vi "DisplayJson.vi"(11 "JSON String In":string="[{\"version\":\"1.0.0\",\"header\":{\"creationDate\":\"2022-06-03T00:00:00\",\"remarks\":\"\",\"serialNumber\":\"98172\",\"productNumber\":\"123021.1804\",\"productType\":\"PAA-9L\",\"pressureType\":2,\"productSeries\":\"9L\",\"compensatedTemperatureRange\":{\"min\":-10.0,\"max\":80.0,\"unit\":4},\"compensatedPressureRange\":{\"min\":0.0,\"max\":0.35,\"unit\":3},\"electricSupply\":{\"magnitude\":1.0,\"unit\":18},\"orderNumber\":9990266,\"orderPosition\":3,\"orderTargetDispatchDate\":\"2022-06-02T00:00:00+00:00\",\"customerName\":\"DemoData Inc.\",\"customerNumber\":12345678,\"customerOrderNumber\":\"Cust-9990266-123\",\"customerReferenceNumber\":\"\",\"customerProductT...") -> ()   [LabVIEW 2017] (continued)
arget\":{\"pressure\":{\"magnitude\":0.03,\"unit\":3},\"temperature\":{\"magnitude\":80.0,\"unit\":4}},\"environment\":{\"pressure\":{\"magnitude\":0.0300006,\"unit\":3},\"temperature\":{\"magnitude\":79.9513,\"unit\":4},\"supply\":{\"magnitude\":1.0,\"unit\":18}},\"raw\":{\"signal\":{\"magnitude\":18.112910598,\"unit\":22},\"bridgeResistance\":{\"magnitude\":4053.922893,\"unit\":28}},\"compensated\":{\"mathematicalModels\":{\"MM0123\":{\"pressure\":{\"output\":{\"magnitude\":0.0300226,\"unit\":3},\"error\":{\"magnitude\":0.0062805229,\"unit\":7}},\"temperature\":{\"output\":{\"magnitude\":80.0426,\"unit\":4},\"error\":{\"magnitude\":0.091262449,\"unit\":4}}}}}},{\"reference\":\"F_12300_XX_0000098765\",\"environmentTarget\":{\"pressure\":{\"magnitude\":0.11,\"unit\":3},\"temperature\":{\"magnitude\":80.0,\"unit\":4}},\"environment\":{\"pressure\":{\"magnitude\":0.110004,\"unit\":3},\"temperature\":{\"magnitude\":79.9513,\"unit\":4},\"supply\":{\"magnitude\":1.0,\"unit\":18}},\"raw\":{\"signal\":{\"magnitude\":30.219828489,\"unit\":22},\"bridgeResistance\":{\"magnitude\":4049.2092548,\"unit\":28}},\"compensated\":{\"mathematicalModels\":{\"MM0123\":{\"pressure\":{\"output\":{\"magnitude\":0.109956,\"unit\":3},\"error\":{\"magnitude\":-0.013573045,\"unit\":7}},\"temperature\":{\"output\":{\"magnitude\":80.0465,\"unit\":4},\"error\":{\"magnitude\":0.095120343,\"unit\":4}}}}}},{\"reference\":\"F_12300_XX_0000098765\",\"environmentTarget\":{\"pressure\":{\"magnitude\":0.19,\"unit\":3},\"temperature\":{\"magnitude\":80.0,\"unit\":4}},\"environment\":{\"pressure\":{\"magnitude\":0.189994,\"unit\":3},\"temperature\":{\"magnitude\":79.9513,\"unit\":4},\"supply\":{\"magnitude\":1.0,\"unit\":18}},\"raw\":{\"signal\":{\"magnitude\":42.312978657,\"unit\":22},\"bridgeResistance\":{\"magnitude\":4044.5861667,\"unit\":28}},\"compensated\":{\"mathematicalModels\":{\"MM0123\":{\"pressure\":{\"output\":{\"magnitude\":0.189999,\"unit\":3},\"error\":{\"magnitude\":0.0015625619,\"unit\":7}},\"temperature\":{\"output\":{\"magnitude\":80.0544,\"unit\":4},\"error\":{\"magnitude\":0.10309475,\"unit\":4}}}}}},{\"reference\":\"F_12300_XX_0000098765\",\"environmentTarget\":{\"pressure\":{\"magnitude\":0.27,\"unit\":3},\"temperature\":{\"magnitude\":80.0,\"unit\":4}},\"environment\":{\"pressure\":{\"magnitude\":0.270001,\"unit\":3},\"temperature\":{\"magnitude\":79.9513,\"unit\":4},\"supply\":{\"magnitude\":1.0,\"unit\":18}},\"raw\":{\"signal\":{\"magnitude\":54.374135615,\"unit\":22},\"bridgeResistance\":{\"magnitude\":4040.0065092,\"unit\":28}},\"compensated\":{\"mathematicalModels\":{\"MM0123\":{\"pressure\":{\"output\":{\"magnitude\":0.270039,\"unit\":3},\"error\":{\"magnitude\":0.01094065,\"unit\":7}},\"temperature\":{\"output\":{\"magnitude\":80.0614,\"unit\":4},\"error\":{\"magnitude\":0.11007026,\"unit\":4}}}}}},{\"reference\":\"F_12300_XX_0000098765\",\"environmentTarget\":{\"pressure\":{\"magnitude\":0.35,\"unit\":3},\"temperature\":{\"magnitude\":80.0,\"unit\":4}},\"environment\":{\"pressure\":{\"magnitude\":0.349998,\"unit\":3},\"temperature\":{\"magnitude\":79.9513,\"unit\":4},\"supply\":{\"magnitude\":1.0,\"unit\":18}},\"raw\":{\"signal\":{\"magnitude\":66.389691162,\"unit\":22},\"bridgeResistance\":{\"magnitude\":4035.4744179,\"unit\":28}},\"compensated\":{\"mathematicalModels\":{\"MM0123\":{\"pressure\":{\"output\":{\"magnitude\":0.349978,\"unit\":3},\"error\":{\"magnitude\":-0.0056827473,\"unit\":7}},\"temperature\":{\"output\":{\"magnitude\":80.0671,\"unit\":4},\"error\":{\"magnitude\":0.11580255,\"unit\":4}}}}}}]},{\"version\":\"1.0.0\",\"header\":{\"creationDate\":\"2022-06-03T00:00:00\",\"remarks\":\"\",\"serialNumber\":\"98062\",\"productNumber\":\"123021.1804\",\"productType\":\"PAA-9L\",\"pressureType\":2,\"productSeries\":\"9L\",\"compensatedTemperatureRange\":{\"min\":-10.0,\"max\":80.0,\"unit\":4},\"compensatedPressureRange\":{\"min\":0.0,\"max\":0.35,\"unit\":3},\"electricSupply\":{\"magnitude\":1.0,\"unit\":18},\"orderNumber\":9990266,\"orderPosition\":3,\"orderTargetDispatchDate\":\"2022-06-02T00:00:00+00:00\",\"customerName\":\"DemoData Inc.\",\"customerNumber\":12345678,\"customerOrderNumber\":\"Cust-9990266-123\",\"customerReferenceNumber\":\"\",\"customerProductType\":\"123021-1804 Rev.AA\"},\"compensationMethods\":{\"mathematicalModels\":{\"MM0123\":{\"modelType\":\"MM0123\",\"productNumber\":\"000000.0000\",\"compensatedTemperatureRange\":{\"min\":-10.0,\"max\":80.0,\"unit\":4},\"compensatedPressureRange\":{\"min\":0.0,\"max\":0.35,\"unit\":3},\"electricSupply\":{\"magnitude\":1.0,\"unit\":18},\"parts\":{\"pressure\":{\"inputs\":[\"Sig\",\"R\"],\"output\":\"P\",\"description\":\"P = f(Sig,R)\",\"coefficients\":[[4.24498616654,-0.00434870646169,1.65645526915E-06,-2.82503980815E-10,1.80574905609E-14],[-0.136709021669,0.000147073956199,-5.65029989332E-08,9.64480704004E-12,-6.18362859613E-16],[4.40289191256E-05,-2.40851139109E-08,1.82732990774E-12,9.42409772251E-16,-1.43118016035E-19]]},\"temperature\":{\"inputs\":[\"R\",\"Sig\"],\"output\":\"T\",\"description\":\"T = f(R,Sig)\",\"coefficients\":[[-8429.66589229,19.4262004834,-0.189958165455],[8.28473398531,-0.0200345175176,0.000205816813801],[-0.00311774743246,7.78515900293E-06,-8.35927190864E-08],[5.30811398776E-07,-1.34715910968E-09,1.50785989149E-11],[-3.40839033724E-11,8.75216679413E-14,-1.01901855741E-15]]}}}}},\"measurements\":[{\"reference\":\"F_12300_XX_0000098765\",\"environmentTarget\":{\"pressure\":{\"magnitude\":0.03,\"unit\":3},\"temperature\":{\"magnitude\":-10.0,\"unit\":4}},\"environment\":{\"pressure\":{\"magnitude\":0.030006,\"unit\":3},\"temperature\":{\"magnitude\":-10.7286,\"unit\":4},\"supply\":{\"magnitude\":1.0,\"unit\":18}},\"raw\":{\"signal\":{\"magnitude\":16.167899598,\"unit\":22},\"bridgeResistance\":{\"magnitude\":3278.97235,\"unit\":28}},\"compensated\":{\"mathematicalModels\":{\"MM0123\":{\"pressure\":{\"output\":{\"magnitude\":0.0300194,\"unit\":3},\"error\":{\"magnitude\":0.003820477,\"unit\":7}},\"temperature\":{\"output\":{\"magnitude\":-10.8437,\"unit\":4},\"error\":{\"magnitude\":-0.11506924,\"unit\":4}}}}}},{\"reference\":\"F_12300_XX_0000098765\",\"environmentTarget\":{\"pressure\":{\"magnitude\":0.11,\"unit\":3},\"temperature\":{\"magnitude\":-10.0,\"unit\":4}},\"environment\":{\"pressure\":{\"magnitude\":0.110008,\"unit\":3},\"temperature\":{\"magnitude\":-10.7286,\"unit\":4},\"supply\":{\"magnitude\":1.0,\"unit\":18}},\"raw\":{\"signal\":{\"magnitude\":28.175220871,\"unit\":22},\"bridgeResistance\":{\"magnitude\":3274.3397417,\"unit\":28}},\"compensated\":{\"mathematicalModels\":{\"MM0123\":{\"pressure\":{\"output\":{\"magnitude\":0.109973,\"unit\":3},\"error\":{\"magnitude\":-0.010122702,\"unit\":7}},\"temperature\":{\"output\":{\"magnitude\":-10.8462,\"unit\":4},\"error\":{\"magnitude\":-0.11753739,\"unit\":4}}}}}},{\"reference\":\"F_12300_XX_0000098765\",\"environmentTarget\":{\"pressure\":{\"magnitude\":0.19,\"unit\":3},\"temperature\":{\"magnitude\":-10.0,\"unit\":4}},\"environment\":{\"pressure\":{\"magnitude\":0.190005,\"unit\":3},\"temperature\":{\"magnitude\":-10.7286,\"unit\":4},\"supply\":{\"magnitude\":1.0,\"unit\":18}},\"raw\":{\"signal\":{\"magnitude\":40.141769614,\"unit\":22},\"bridgeResistance\":{\"magnitude\":3269.8255782,\"unit\":28}},\"compensated\":{\"mathematicalModels\":{\"MM0123\":{\"pressure\":{\"output\":{\"magnitude\":0.190013,\"unit\":3},\"error\":{\"magnitude\":0.0022029902,\"unit\":7}},\"temperature\":{\"output\":{\"magnitude\":-10.8464,\"unit\":4},\"error\":{\"magnitude\":-0.11774787,\"unit\":4}}}}}},{\"reference\":\"F_12300_XX_0000098765\",\"environmentTarget\":{\"pressure\":{\"magnitude\":0.27,\"unit\":3},\"temperature\":{\"magnitude\":-10.0,\"unit\":4}},\"environment\":{\"pressure\":{\"magnitude\":0.270008,\"unit\":3},\"temperature\":{\"magnitude\":-10.7286,\"unit\":4},\"supply\":{\"magnitude\":1.0,\"unit\":18}},\"raw\":{\"signal\":{\"magnitude\":52.052658113,\"unit\":22},\"bridgeResistance\":{\"magnitude\":3265.4291158,\"unit\":28}},\"compensated\":{\"mathematicalModels\":{\"MM0123\":{\"pressure\":{\"output\":{\"magnitude\":0.270043,\"unit\":3},\"error\":{\"magnitude\":0.0098634549,\"unit\":7}},\"temperature\":{\"output\":{\"magnitude\":-10.8462,\"unit\":4},\"error\":{\"magnitude\":-0.11753424,\"unit\":4}}}}}},{\"reference\":\"F_12300_XX_0000098765\",\"environmentTarget\":{\"pressure\":{\"magnitude\":0.35,\"unit\":3},\"temperature\":{\"magnitude\":-10.0,\"unit\":4}},\"environment\":{\"pressure\":{\"magnitude\":0.350001,\"unit\":3},\"temperature\":{\"magnitude\":-10.7286,\"unit\":4},\"supply\":{\"magnitude\":1.0,\"unit\":18}},\"raw\":{\"signal\":{\"magnitude\":63.897706655,\"unit\":22},\"bridgeResistance\":{\"magnitude\":3261.1318651,\"unit\":28}},\"compensated\":{\"mathematicalModels\":{\"MM0123\":{\"pressure\":{\"output\":{\"magnitude\":0.349995,\"unit\":3},\"error\":{\"magnitude\":-0.0017233202,\"unit\":7}},\"temperature\":{\"output\":{\"magnitude\":-10.8497,\"unit\":4},\"error\":{\"magnitude\":-0.12110753,\"unit\":4}}}}}},{\"reference\":\"F_12300_XX_0000098765\",\"environmentTarget\":{\"pressure\":{\"magnitude\":0.03,\"unit\":3},\"temperature\":{\"magnitude\":0.0,\"unit\":4}},\"environment\":{\"pressure\":{\"magnitude\":0.0300032,\"unit\":3},\"temperature\":{\"magnitude\":-0.629962,\"unit\":4},\"supply\":{\"magnitude\":1.0,\"unit\":18}},\"raw\":{\"signal\":{\"magnitude\":16.623830617,\"unit\":22},\"bridgeResistance\":{\"magnitude\":3347.8748473,\"unit\":28}},\"compensated\":{\"mathematicalModels\":{\"MM0123\":{\"pressure\":{\"output\":{\"magnitude\":0.0300186,\"unit\":3},\"error\":{\"magnitude\":0.0044065173,\"unit\":7}},\"temperature\":{\"output\":{\"magnitude\":-0.743773,\"unit\":4},\"error\":{\"magnitude\":-0.11381103,\"unit\":4}}}}}},{\"reference\":\"F_12300_XX_0000098765\",\"environmentTarget\":{\"pressure\":{\"magnitude\":0.11,\"unit\":3},\"temperature\":{\"magnitude\":0.0,\"unit\":4}},\"environment\":{\"pressure\":{\"magnitude\":0.110005,\"unit\":3},\"temperature\":{\"magnitude\":-0.629962,\"unit\":4},\"supply\":{\"magnitude\":1.0,\"unit\":18}},\"raw\":{\"signal\":{\"magnitude\":28.598303294,\"unit\":22},\"bridgeResistance\":{\"magnitude\":3343.279329,\"unit\":28}},\"compensated\":{\"mathematicalModels\":{\"MM0123\":{\"pressure\":{\"output\":{\"magnitude\":0.109969,\"unit\":3},\"error\":{\"magnitude\":-0.010291145,\"unit\":7}},\"temperature\":{\"output\":{\"magnitude\":-0.747222,\"unit\":4},\"error\":{\"magnitude\":-0.11726057,\"unit\":4}}}}}},{\"reference\":\"F_12300_XX_0000098765\",\"environmentTarget\":{\"pressure\":{\"magnitude\":0.19,\"unit\":3},\"temperature\":{\"magnitude\":0.0,\"unit\":4}},\"environment\":{\"pressure\":{\"magnitude\":0.190007,\"unit\":3},\"temperature\":{\"magnitude\":-0.629962,\"unit\":4},\"supply\":{\"magnitude\":1.0,\"unit\":18}},\"raw\":{\"signal\":{\"magnitude\":40.534914808,\"unit\":22},\"bridgeResistance\":{\"magnitude\":3338.7917735,\"unit\":28}},\"compensated\":{\"mathematicalModels\":{\"MM0123\":{\"pressure\":{\"output\":{\"magnitude\":0.190008,\"unit\":3},\"error\":{\"magnitude\":0.00028916783,\"unit\":7}},\"temperature\":{\"output\":{\"magnitude\":-0.74744,\"unit\":4},\"error\":{\"magnitude\":-0.11747789,\"unit\":4}}}}}},{\"reference\":\"F_12300_XX_0000098765\",\"environmentTarget\":{\"pressure\":{\"magnitude\":0.27,\"unit\":3},\"temperature\":{\"magnitude\":0.0,\"unit\":4}},\"environment\":{\"pressure\":{\"magnitude\":0.269999,\"unit\":3},\"temperature\":{\"magnitude\":-0.629962,\"unit\":4},\"supply\":{\"magnitude\":1.0,\"unit\":18}},\"raw\":{\"signal\":{\"magnitude\":52.415254612,\"unit\":22},\"bridgeResistance\":{\"magnitude\":3334.362312,\"unit\":28}},\"compensated\":{\"mathematicalModels\":{\"MM0123\":{\"pressure\":{\"output\":{\"magnitude\":0.270016,\"unit\":3},\"error\":{\"magnitude\":0.0047200097,\"unit\":7}},\"temperature\":{\"output\":{\"magnitude\":-0.752861,\"unit\":4},\"error\":{\"magnitude\":-0.12289898,\"unit\":4}}}}}},{\"reference\":\"F_12300_XX_0000098765\",\"environmentTarget\":{\"pressure\":{\"magnitude\":0.35,\"unit\":3},\"temperature\":{\"magnitude\":0.0,\"unit\":4}},\"environment\":{\"pressure\":{\"magnitude\":0.350007,\"unit\":3},\"temperature\":{\"magnitude\":-0.629962,\"unit\":4},\"supply\":{\"magnitude\":1.0,\"unit\":18}},\"raw\":{\"signal\":{\"magnitude\":64.236943105,\"unit\":22},\"bridgeResistance\":{\"magnitude\":3330.0559863,\"unit\":28}},\"compensated\":{\"mathematicalModels\":{\"MM0123\":{\"pressure\":{\"output\":{\"magnitude\":0.349973,\"unit\":3},\"error\":{\"magnitude\":-0.0097175853,\"unit\":7}},\"temperature\":{\"output\":{\"magnitude\":-0.754914,\"unit\":4},\"error\":{\"magnitude\":-0.12495178,\"unit\":4}}}}}},{\"reference\":\"F_12300_XX_0000098765\",\"environmentTarget\":{\"pressure\":{\"magnitude\":0.03,\"unit\":3},\"temperature\":{\"magnitude\":20.0,\"unit\":4}},\"environment\":{\"pressure\":{\"magnitude\":0.0299948,\"unit\":3},\"temperature\":{\"magnitude\":19.5509,\"unit\":4},\"supply\":{\"magnitude\":1.0,\"unit\":18}},\"raw\":{\"signal\":{\"magnitude\":17.582834891,\"unit\":22},\"bridgeResistance\":{\"magnitude\":3503.2026052,\"unit\":28}},\"compensated\":{\"mathematicalModels\":{\"MM0123\":{\"pressure\":{\"output\":{\"magnitude\":0.0300099,\"unit\":3},\"error\":{\"magnitude\":0.004308579,\"unit\":7}},\"temperature\":{\"output\":{\"magnitude\":19.5413,\"unit\":4},\"error\":{\"magnitude\":-0.009571961,\"unit\":4}}}}}},{\"reference\":\"F_12300_XX_0000098765\",\"environmentTarget\":{\"pressure\":{\"magnitude\":0.11,\"unit\":3},\"temperature\":{\"magnitude\":20.0,\"unit\":4}},\"environment\":{\"pressure\":{\"magnitude\":0.109994,\"unit\":3},\"temperature\":{\"magnitude\":19.5509,\"unit\":4},\"supply\":{\"magnitude\":1.0,\"unit\":18}},\"raw\":{\"signal\":{\"magnitude\":29.550682095,\"unit\":22},\"bridgeResistance\":{\"magnitude\":3498.58799,\"unit\":28}},\"compensated\":{\"mathematicalModels\":{\"MM0123\":{\"pressure\":{\"output\":{\"magnitude\":0.109966,\"unit\":3},\"error\":{\"magnitude\":-0.008013191,\"unit\":7}},\"temperature\":{\"output\":{\"magnitude\":19.5351,\"unit\":4},\"error\":{\"magnitude\":-0.015746182,\"unit\":4}}}}}},{\"reference\":\"F_12300_XX_0000098765\",\"environmentTarget\":{\"pressure\":{\"magnitude\":0.19,\"unit\":3},\"temperature\":{\"magnitude\":20.0,\"unit\":4}},\"environment\":{\"pressure\":{\"magnitude\":0.19,\"unit\":3},\"temperature\":{\"magnitude\":19.5509,\"unit\":4},\"supply\":{\"magnitude\":1.0,\"unit\":18}},\"raw\":{\"signal\":{\"magnitude\":41.485081135,\"unit\":22},\"bridgeResistance\":{\"magnitude\":3494.0870258,\"unit\":28}},\"compensated\":{\"mathematicalModels\":{\"MM0123\":{\"pressure\":{\"output\":{\"magnitude\":0.190006,\"unit\":3},\"error\":{\"magnitude\":0.0016759146,\"unit\":7}},\"temperature\":{\"output\":{\"magnitude\":19.5339,\"unit\":4},\"error\":{\"magnitude\":-0.016980767,\"unit\":4}}}}}},{\"reference\":\"F_12300_XX_0000098765\",\"environmentTarget\":{\"pressure\":{\"magnitude\":0.27,\"unit\":3},\"temperature\":{\"magnitude\":20.0,\"unit\":4}},\"environment\":{\"pressure\":{\"magnitude\":0.269991,\"unit\":3},\"temperature\":{\"magnitude\":19.5509,\"unit\":4},\"supply\":{\"magnitude\":1.0,\"unit\":18}},\"raw\":{\"signal\":{\"magnitude\":53.37070629,\"unit\":22},\"bridgeResistance\":{\"magnitude\":3489.6192286,\"unit\":28}},\"compensated\":{\"mathematicalModels\":{\"MM0123\":{\"pressure\":{\"output\":{\"magnitude\":0.270031,\"unit\":3},\"error\":{\"magnitude\":0.011358778,\"unit\":7}},\"temperature\":{\"output\":{\"magnitude\":19.5271,\"unit\":4},\"error\":{\"magnitude\":-0.0237925,\"unit\":4}}}}}},{\"reference\":\"F_12300_XX_0000098765\",\"environmentTarget\":{\"pressure\":{\"magnitude\":0.35,\"unit\":3},\"temperature\":{\"magnitude\":20.0,\"unit\":4}},\"environment\":{\"pressure\":{\"magnitude\":0.350002,\"unit\":3},\"temperature\":{\"magnitude\":19.5509,\"unit\":4},\"supply\":{\"magnitude\":1.0,\"unit\":18}},\"raw\":{\"signal\":{\"magnitude\":65.203270025,\"unit\":22},\"bridgeResistance\":{\"magnitude\":3485.2648231,\"unit\":28}},\"compensated\":{\"mathematicalModels\":{\"MM0123\":{\"pressure\":{\"output\":{\"magnitude\":0.350008,\"unit\":3},\"error\":{\"magnitude\":0.0016539591,\"unit\":7}},\"temperature\":{\"output\":{\"magnitude\":19.5242,\"unit\":4},\"error\":{\"magnitude\":-0.026645966,\"unit\":4}}}}}},{\"reference\":\"F_12300_XX_0000098765\",\"environmentTarget\":{\"pressure\":{\"magnitude\":0.03,\"unit\":3},\"temperature\":{\"magnitude\":40.0,\"unit\":4}},\"environment\":{\"pressure\":{\"magnitude\":0.0300084,\"unit\":3},\"temperature\":{\"magnitude\":39.7284,\"unit\":4},\"supply\":{\"magnitude\":1.0,\"unit\":18}},\"raw\":{\"signal\":{\"magnitude\":18.627411057,\"unit\":22},\"bridgeResistance\":{\"magnitude\":3679.0495206,\"unit\":28}},\"compensated\":{\"mathematicalModels\":{\"MM0123\":{\"pressure\":{\"output\":{\"magnitude\":0.0300252,\"unit\":3},\"error\":{\"magnitude\":0.004810232,\"unit\":7}},\"temperature\":{\"output\":{\"magnitude\":39.7236,\"unit\":4},\"error\":{\"magnitude\":-0.0048319572,\"unit\":4}}}}}},{\"reference\":\"F_12300_XX_0000098765\",\"environmentTarget\":{\"pressure\":{\"magnitude\":0.11,\"unit\":3},\"temperature\":{\"magnitude\":40.0,\"unit\":4}},\"environment\":{\"pressure\":{\"magnitude\":0.110007,\"unit\":3},\"temperature\":{\"magnitude\":39.7284,\"unit\":4},\"supply\":{\"magnitude\":1.0,\"unit\":18}},\"raw\":{\"signal\":{\"magnitude\":30.651007346,\"unit\":22},\"bridgeResistance\":{\"magnitude\":3674.4400569,\"unit\":28}},\"compensated\":{\"mathematicalModels\":{\"MM0123\":{\"pressure\":{\"output\":{\"magnitude\":0.109971,\"unit\":3},\"error\":{\"magnitude\":-0.010377962,\"unit\":7}},\"temperature\":{\"output\":{\"magnitude\":39.7252,\"unit\":4},\"error\":{\"magnitude\":-0.0031891045,\"unit\":4}}}}}},{\"reference\":\"F_12300_XX_0000098765\",\"environmentTarget\":{\"pressure\":{\"magnitude\":0.19,\"unit\":3},\"temperature\":{\"magnitude\":40.0,\"unit\":4}},\"environment\":{\"pressure\":{\"magnitude\":0.190003,\"unit\":3},\"temperature\":{\"magnitude\":39.7284,\"unit\":4},\"supply\":{\"magnitude\":1.0,\"unit\":18}},\"raw\":{\"signal\":{\"magnitude\":42.645937338,\"unit\":22},\"bridgeResistance\":{\"magnitude\":3669.8548566,\"unit\":28}},\"compensated\":{\"mathematicalModels\":{\"MM0123\":{\"pressure\":{\"output\":{\"magnitude\":0.190003,\"unit\":3},\"error\":{\"magnitude\":0.00012410203,\"unit\":7}},\"temperature\":{\"output\":{\"magnitude\":39.7218,\"unit\":4},\"error\":{\"magnitude\":-0.0066113459,\"unit\":4}}}}}},{\"reference\":\"F_12300_XX_0000098765\",\"environmentTarget\":{\"pressure\":{\"magnitude\":0.27,\"unit\":3},\"temperature\":{\"magnitude\":40.0,\"unit\":4}},\"environment\":{\"pressure\":{\"magnitude\":0.269997,\"unit\":3},\"temperature\":{\"magnitude\":39.7284,\"unit\":4},\"supply\":{\"magnitude\":1.0,\"unit\":18}},\"raw\":{\"signal\":{\"magnitude\":54.596933139,\"unit\":22},\"bridgeResistance\":{\"magnitude\":3665.3639897,\"unit\":28}},\"compensated\":{\"mathematicalModels\":{\"MM0123\":{\"pressure\":{\"output\":{\"magnitude\":0.270019,\"unit\":3},\"error\":{\"magnitude\":0.0062796257,\"unit\":7}},\"temperature\":{\"output\":{\"magnitude\":39.7203,\"unit\":4},\"error\":{\"magnitude\":-0.0081685864,\"unit\":4}}}}}},{\"reference\":\"F_12300_XX_0000098765\",\"environmentTarget\":{\"pressure\":{\"magnitude\":0.35,\"unit\":3},\"temperature\":{\"magnitude\":40.0,\"unit\":4}},\"environment\":{\"pressure\":{\"magnitude\":0.350004,\"unit\":3},\"temperature\":{\"magnitude\":39.7284,\"unit\":4},\"supply\":{\"magnitude\":1.0,\"unit\":18}},\"raw\":{\"signal\":{\"magnitude\":66.497713991,\"unit\":22},\"bridgeResistance\":{\"magnitude\":3660.974451,\"unit\":28}},\"compensated\":{\"mathematicalModels\":{\"MM0123\":{\"pressure\":{\"output\":{\"magnitude\":0.349974,\"unit\":3},\"error\":{\"magnitude\":-0.0085700125,\"unit\":7}},\"temperature\":{\"output\":{\"magnitude\":39.721,\"unit\":4},\"error\":{\"magnitude\":-0.0073826446,\"unit\":4}}}}}},{\"reference\":\"F_12300_XX_0000098765\",\"environmentTarget\":{\"pressure\":{\"magnitude\":0.03,\"unit\":3},\"temperature\":{\"magnitude\":60.0,\"unit\":4}},\"environment\":{\"pressure\":{\"magnitude\":0.0299893,\"unit\":3},\"temperature\":{\"magnitude\":59.8651,\"unit\":4},\"supply\":{\"magnitude\":1.0,\"unit\":18}},\"raw\":{\"signal\":{\"magnitude\":19.781683569,\"unit\":22},\"bridgeResistance\":{\"magnitude\":3872.1157928,\"unit\":28}},\"compensated\":{\"mathematicalModels\":{\"MM0123\":{\"pressure\":{\"output\":{\"magnitude\":0.030007,\"unit\":3},\"error\":{\"magnitude\":0.0050456891,\"unit\":7}},\"temperature\":{\"output\":{\"magnitude\":59.9294,\"unit\":4},\"error\":{\"magnitude\":0.064229229,\"unit\":4}}}}}},{\"reference\":\"F_12300_XX_0000098765\",\"environmentTarget\":{\"pressure\":{\"magnitude\":0.11,\"unit\":3},\"temperature\":{\"magnitude\":60.0,\"unit\":4}},\"environment\":{\"pressure\":{\"magnitude\":0.110007,\"unit\":3},\"temperature\":{\"magnitude\":59.8651,\"unit\":4},\"supply\":{\"magnitude\":1.0,\"unit\":18}},\"raw\":{\"signal\":{\"magnitude\":31.905431169,\"unit\":22},\"bridgeResistance\":{\"magnitude\":3867.4425868,\"unit\":28}},\"compensated\":{\"mathematicalModels\":{\"MM0123\":{\"pressure\":{\"output\":{\"magnitude\":0.109971,\"unit\":3},\"error\":{\"magnitude\":-0.010382341,\"unit\":7}},\"temperature\":{\"output\":{\"magnitude\":59.9314,\"unit\":4},\"error\":{\"magnitude\":0.066286714,\"unit\":4}}}}}},{\"reference\":\"F_12300_XX_0000098765\",\"environmentTarget\":{\"pressure\":{\"magnitude\":0.19,\"unit\":3},\"temperature\":{\"magnitude\":60.0,\"unit\":4}},\"environment\":{\"pressure\":{\"magnitude\":0.189997,\"unit\":3},\"temperature\":{\"magnitude\":59.8651,\"unit\":4},\"supply\":{\"magnitude\":1.0,\"unit\":18}},\"raw\":{\"signal\":{\"magnitude\":44.002565704,\"unit\":22},\"bridgeResistance\":{\"magnitude\":3862.8300303,\"unit\":28}},\"compensated\":{\"mathematicalModels\":{\"MM0123\":{\"pressure\":{\"output\":{\"magnitude\":0.190001,\"unit\":3},\"error\":{\"magnitude\":0.0010387379,\"unit\":7}},\"temperature\":{\"output\":{\"magnitude\":59.9345,\"unit\":4},\"error\":{\"magnitude\":0.069326144,\"unit\":4}}}}}},{\"reference\":\"F_12300_XX_0000098765\",\"environmentTarget\":{\"pressure\":{\"magnitude\":0.27,\"unit\":3},\"temperature\":{\"magnitude\":60.0,\"unit\":4}},\"environment\":{\"pressure\":{\"magnitude\":0.270006,\"unit\":3},\"temperature\":{\"magnitude\":59.8651,\"unit\":4},\"supply\":{\"magnitude\":1.0,\"unit\":18}},\"raw\":{\"signal\":{\"magnitude\":56.064516352,\"unit\":22},\"bridgeResistance\":{\"magnitude\":3858.2425119,\"unit\":28}},\"compensated\":{\"mathematicalModels\":{\"MM0123\":{\"pressure\":{\"output\":{\"magnitude\":0.270043,\"unit\":3},\"error\":{\"magnitude\":0.010491266,\"unit\":7}},\"temperature\":{\"output\":{\"magnitude\":59.9344,\"unit\":4},\"error\":{\"magnitude\":0.06926337,\"unit\":4}}}}}},{\"reference\":\"F_12300_XX_0000098765\",\"environmentTarget\":{\"pressure\":{\"magnitude\":0.35,\"unit\":3},\"temperature\":{\"magnitude\":60.0,\"unit\":4}},\"environment\":{\"pressure\":{\"magnitude\":0.349994,\"unit\":3},\"temperature\":{\"magnitude\":59.8651,\"unit\":4},\"supply\":{\"magnitude\":1.0,\"unit\":18}},\"raw\":{\"signal\":{\"magnitude\":68.074620907,\"unit\":22},\"bridgeResistance\":{\"magnitude\":3853.7631514,\"unit\":28}},\"compensated\":{\"mathematicalModels\":{\"MM0123\":{\"pressure\":{\"output\":{\"magnitude\":0.349982,\"unit\":3},\"error\":{\"magnitude\":-0.0033827747,\"unit\":7}},\"temperature\":{\"output\":{\"magnitude\":59.9389,\"unit\":4},\"error\":{\"magnitude\":0.073681518,\"unit\":4}}}}}},{\"reference\":\"F_12300_XX_0000098765\",\"environmentTarget\":{\"pressure\":{\"magnitude\":0.03,\"unit\":3},\"temperature\":{\"magnitude\":80.0,\"unit\":4}},\"environment\":{\"pressure\":{\"magnitude\":0.0300004,\"unit\":3},\"temperature\":{\"magnitude\":79.9513,\"unit\":4},\"supply\":{\"magnitude\":1.0,\"unit\":18}},\"raw\":{\"signal\":{\"magnitude\":21.08114189,\"unit\":22},\"bridgeResistance\":{\"magnitude\":4079.4822134,\"unit\":28}},\"compensated\":{\"mathematicalModels\":{\"MM0123\":{\"pressure\":{\"output\":{\"magnitude\":0.0300223,\"unit\":3},\"error\":{\"magnitude\":0.0062645074,\"unit\":7}},\"temperature\":{\"output\":{\"magnitude\":80.0522,\"unit\":4},\"error\":{\"magnitude\":0.10089745,\"unit\":4}}}}}},{\"reference\":\"F_12300_XX_0000098765\",\"environmentTarget\":{\"pressure\":{\"magnitude\":0.11,\"unit\":3},\"temperature\":{\"magnitude\":80.0,\"unit\":4}},\"environment\":{\"pressure\":{\"magnitude\":0.110007,\"unit\":3},\"temperature\":{\"magnitude\":79.9513,\"unit\":4},\"supply\":{\"magnitude\":1.0,\"unit\":18}},\"raw\":{\"signal\":{\"magnitude\":33.327527613,\"unit\":22},\"bridgeResistance\":{\"magnitude\":4074.7150768,\"unit\":28}},\"compensated\":{\"mathematicalModels\":{\"MM0123\":{\"pressure\":{\"output\":{\"magnitude\":0.109961,\"unit\":3},\"error\":{\"magnitude\":-0.013118302,\"unit\":7}},\"temperature\":{\"output\":{\"magnitude\":80.0563,\"unit\":4},\"error\":{\"magnitude\":0.10491776,\"unit\":4}}}}}},{\"reference\":\"F_12300_XX_0000098765\",\"environmentTarget\":{\"pressure\":{\"magnitude\":0.19,\"unit\":3},\"temperature\":{\"magnitude\":80.0,\"unit\":4}},\"environment\":{\"pressure\":{\"magnitude\":0.190006,\"unit\":3},\"temperature\":{\"magnitude\":79.9513,\"unit\":4},\"supply\":{\"magnitude\":1.0,\"unit\":18}},\"raw\":{\"signal\":{\"magnitude\":45.560736744,\"unit\":22},\"bridgeResistance\":{\"magnitude\":4070.040075,\"unit\":28}},\"compensated\":{\"mathematicalModels\":{\"MM0123\":{\"pressure\":{\"output\":{\"magnitude\":0.190014,\"unit\":3},\"error\":{\"magnitude\":0.0023306954,\"unit\":7}},\"temperature\":{\"output\":{\"magnitude\":80.0637,\"unit\":4},\"error\":{\"magnitude\":0.11233408,\"unit\":4}}}}}},{\"reference\":\"F_12300_XX_0000098765\",\"environmentTarget\":{\"pressure\":{\"magnitude\":0.27,\"unit\":3},\"temperature\":{\"magnitude\":80.0,\"unit\":4}},\"environment\":{\"pressure\":{\"magnitude\":0.270004,\"unit\":3},\"temperature\":{\"magnitude\":79.9513,\"unit\":4},\"supply\":{\"magnitude\":1.0,\"unit\":18}},\"raw\":{\"signal\":{\"magnitude\":57.758426133,\"unit\":22},\"bridgeResistance\":{\"magnitude\":4065.431203,\"unit\":28}},\"compensated\":{\"mathematicalModels\":{\"MM0123\":{\"pressure\":{\"output\":{\"magnitude\":0.270038,\"unit\":3},\"error\":{\"magnitude\":0.0098415905,\"unit\":7}},\"temperature\":{\"output\":{\"magnitude\":80.0718,\"unit\":4},\"error\":{\"magnitude\":0.1204067,\"unit\":4}}}}}},{\"reference\":\"F_12300_XX_0000098765\",\"environmentTarget\":{\"pressure\":{\"magnitude\":0.35,\"unit\":3},\"temperature\":{\"magnitude\":80.0,\"unit\":4}},\"environment\":{\"pressure\":{\"magnitude\":0.349997,\"unit\":3},\"temperature\":{\"magnitude\":79.9513,\"unit\":4},\"supply\":{\"magnitude\":1.0,\"unit\":18}},\"raw\":{\"signal\":{\"magnitude\":69.911761084,\"unit\":22},\"bridgeResistance\":{\"magnitude\":4060.8489395,\"unit\":28}},\"compensated\":{\"mathematicalModels\":{\"MM0123\":{\"pressure\":{\"output\":{\"magnitude\":0.349979,\"unit\":3},\"error\":{\"magnitude\":-0.0050469422,\"unit\":7}},\"temperature\":{\"output\":{\"magnitude\":80.0769,\"unit\":4},\"error\":{\"magnitude\":0.12557462,\"unit\":4}}}}}}]},{\"version\":\"1.0.0\",\"header\":{\"creationDate\":\"2022-06-03T00:00:00\",\"remarks\":\"\",\"serialNumber\":\"98061\",\"productNumber\":\"123021.1804\",\"productType\":\"PAA-9L\",\"pressureType\":2,\"productSeries\":\"9L\",\"compensatedTemperatureRange\":{\"min\":-10.0,\"max\":80.0,\"unit\":4},\"compensatedPressureRange\":{\"min\":0.0,\"max\":0.35,\"unit\":3},\"electricSupply\":{\"magnitude\":1.0,\"unit\":18},\"orderNumber\":9990266,\"orderPosition\":3,\"orderTargetDispatchDate\":\"2022-06-02T00:00:00+00:00\",\"customerName\":\"DemoData Inc.\",\"customerNumber\":12345678,\"customerOrderNumber\":\"Cust-9990266-123\",\"customerReferenceNumber\":\"\",\"customerProductType\":\"123021-1804 Rev.AA\"},\"compensationMethods\":{\"mathematicalModels\":{\"MM0123\":{\"modelType\":\"MM0123\",\"productNumber\":\"000000.0000\",\"compensatedTemperatureRange\":{\"min\":-10.0,\"max\":80.0,\"unit\":4},\"compensatedPressureRange\":{\"min\":0.0,\"max\":0.35,\"unit\":3},\"electricSupply\":{\"magnitude\":1.0,\"unit\":18},\"parts\":{\"pressure\":{\"inputs\":[\"Sig\",\"R\"],\"output\":\"P\",\"description\":\"P = f(Sig,R)\",\"coefficients\":[[5.00925110961,-0.00515329331367,1.97271220321E-06,-3.37996868347E-10,2.17096400747E-14],[-0.165789433327,0.000178623781506,-6.90954943014E-08,1.18757696952E-11,-7.66451619613E-16],[0.000293446391784,-2.94257716964E-07,1.11322573227E-10,-1.87308929289E-14,1.17878193312E-18]]},\"temperature\":{\"inputs\":[\"R\",\"Sig\"],\"output\":\"T\",\"description\":\"T = f(R,Sig)\",\"coefficients\":[[-8589.2709499,24.44652037,-0.248018222581],[8.46864340333,-0.0255801989632,0.000269636482368],[-0.00319657436096,1.00748923352E-05,-1.09832958618E-07],[5.4569791363E-07,-1.7660238032E-09,1.98610693294E-11],[-3.51301587845E-11,1.16168057332E-13,-1.34500232891E-15]]}}}}},\"measurements\":[{\"reference\":\"F_12300_XX_0000098765\",\"environmentTarget\":{\"pressure\":{\"magnitude\":0.03,\"unit\":3},\"temperature\":{\"magnitude\":-10.0,\"unit\":4}},\"environment\":{\"pressure\":{\"magnitude\":0.030008,\"unit\":3},\"temperature\":{\"magnitude\":-10.7286,\"unit\":4},\"supply\":{\"magnitude\":1.0,\"unit\":18}},\"raw\":{\"signal\":{\"magnitude\":16.070182523,\"unit\":22},\"bridgeResistance\":{\"magnitude\":3273.9892432,\"unit\":28}},\"compensated\":{\"mathematicalModels\":{\"MM0123\":{\"pressure\":{\"output\":{\"magnitude\":0.0300163,\"unit\":3},\"error\":{\"magnitude\":0.0023720538,\"unit\":7}},\"temperature\":{\"output\":{\"magnitude\":-10.8444,\"unit\":4},\"error\":{\"magnitude\":-0.11574486,\"unit\":4}}}}}},{\"reference\":\"F_12300_XX_0000098765\",\"environmentTarget\":{\"pressure\":{\"magnitude\":0.11,\"unit\":3},\"temperature\":{\"magnitude\":-10.0,\"unit\":4}},\"environment\":{\"pressure\":{\"magnitude\":0.110005,\"unit\":3},\"temperature\":{\"magnitude\":-10.7286,\"unit\":4},\"supply\":{\"magnitude\":1.0,\"unit\":18}},\"raw\":{\"signal\":{\"magnitude\":27.221301309,\"unit\":22},\"bridgeResistance\":{\"magnitude\":3269.7406543,\"unit\":28}},\"compensated\":{\"mathematicalModels\":{\"MM0123\":{\"pressure\":{\"output\":{\"magnitude\":0.109979,\"unit\":3},\"error\":{\"magnitude\":-0.0075140673,\"unit\":7}},\"temperature\":{\"output\":{\"magnitude\":-10.8466,\"unit\":4},\"error\":{\"magnitude\":-0.11792636,\"unit\":4}}}}}},{\"reference\":\"F_12300_XX_0000098765\",\"environmentTarget\":{\"pressure\":{\"magnitude\":0.19,\"unit\":3},\"temperature\":{\"magnitude\":-10.0,\"unit\":4}},\"environment\":{\"pressure\":{\"magnitude\":0.190004,\"unit\":3},\"temperature\":{\"magnitude\":-10.7286,\"unit\":4},\"supply\":{\"magnitude\":1.0,\"unit\":18}},\"raw\":{\"signal\":{\"magnitude\":38.338710549,\"unit\":22},\"bridgeResistance\":{\"magnitude\":3265.6086334,\"unit\":28}},\"compensated\":{\"mathematicalModels\":{\"MM0123\":{\"pressure\":{\"output\":{\"magnitude\":0.190012,\"unit\":3},\"error\":{\"magnitude\":0.0022893324,\"unit\":7}},\"temperature\":{\"output\":{\"magnitude\":-10.8458,\"unit\":4},\"error\":{\"magnitude\":-0.11712251,\"unit\":4}}}}}},{\"reference\":\"F_12300_XX_0000098765\",\"environmentTarget\":{\"pressure\":{\"magnitude\":0.27,\"unit\":3},\"temperature\":{\"magnitude\":-10.0,\"unit\":4}},\"environment\":{\"pressure\":{\"magnitude\":0.270006,\"unit\":3},\"temperature\":{\"magnitude\":-10.7286,\"unit\":4},\"supply\":{\"magnitude\":1.0,\"unit\":18}},\"raw\":{\"signal\":{\"magnitude\":49.410196661,\"unit\":22},\"bridgeResistance\":{\"magnitude\":3261.5815393,\"unit\":28}},\"compensated\":{\"mathematicalModels\":{\"MM0123\":{\"pressure\":{\"output\":{\"magnitude\":0.270032,\"unit\":3},\"error\":{\"magnitude\":0.0073468171,\"unit\":7}},\"temperature\":{\"output\":{\"magnitude\":-10.8451,\"unit\":4},\"error\":{\"magnitude\":-0.11645166,\"unit\":4}}}}}},{\"reference\":\"F_12300_XX_0000098765\",\"environmentTarget\":{\"pressure\":{\"magnitude\":0.35,\"unit\":3},\"temperature\":{\"magnitude\":-10.0,\"unit\":4}},\"environment\":{\"pressure\":{\"magnitude\":0.350003,\"unit\":3},\"temperature\":{\"magnitude\":-10.7286,\"unit\":4},\"supply\":{\"magnitude\":1.0,\"unit\":18}},\"raw\":{\"signal\":{\"magnitude\":60.429920438,\"unit\":22},\"bridgeResistance\":{\"magnitude\":3257.6500273,\"unit\":28}},\"compensated\":{\"mathematicalModels\":{\"MM0123\":{\"pressure\":{\"output\":{\"magnitude\":0.349998,\"unit\":3},\"error\":{\"magnitude\":-0.0015064625,\"unit\":7}},\"temperature\":{\"output\":{\"magnitude\":-10.8471,\"unit\":4},\"error\":{\"magnitude\":-0.1184381,\"unit\":4}}}}}},{\"reference\":\"F_12300_XX_0000098765\",\"environmentTarget\":{\"pressure\":{\"magnitude\":0.03,\"unit\":3},\"temperature\":{\"magnitude\":0.0,\"unit\":4}},\"environment\":{\"pressure\":{\"magnitude\":0.0299996,\"unit\":3},\"temperature\":{\"magnitude\":-0.629962,\"unit\":4},\"supply\":{\"magnitude\":1.0,\"unit\":18}},\"raw\":{\"signal\":{\"magnitude\":16.537892175,\"unit\":22},\"bridgeResistance\":{\"magnitude\":3342.6610145,\"unit\":28}},\"compensated\":{\"mathematicalModels\":{\"MM0123\":{\"pressure\":{\"output\":{\"magnitude\":0.0300107,\"unit\":3},\"error\":{\"magnitude\":0.0031672192,\"unit\":7}},\"temperature\":{\"output\":{\"magnitude\":-0.74463,\"unit\":4},\"error\":{\"magnitude\":-0.11466817,\"unit\":4}}}}}},{\"reference\":\"F_12300_XX_0000098765\",\"environmentTarget\":{\"pressure\":{\"magnitude\":0.11,\"unit\":3},\"temperature\":{\"magnitude\":0.0,\"unit\":4}},\"environment\":{\"pressure\":{\"magnitude\":0.11,\"unit\":3},\"temperature\":{\"magnitude\":-0.629962,\"unit\":4},\"supply\":{\"magnitude\":1.0,\"unit\":18}},\"raw\":{\"signal\":{\"magnitude\":27.656903859,\"unit\":22},\"bridgeResistance\":{\"magnitude\":3338.4544626,\"unit\":28}},\"compensated\":{\"mathematicalModels\":{\"MM0123\":{\"pressure\":{\"output\":{\"magnitude\":0.109973,\"unit\":3},\"error\":{\"magnitude\":-0.007720313,\"unit\":7}},\"temperature\":{\"output\":{\"magnitude\":-0.74751,\"unit\":4},\"error\":{\"magnitude\":-0.11754802,\"unit\":4}}}}}},{\"reference\":\"F_12300_XX_0000098765\",\"environmentTarget\":{\"pressure\":{\"magnitude\":0.19,\"unit\":3},\"temperature\":{\"magnitude\":0.0,\"unit\":4}},\"environment\":{\"pressure\":{\"magnitude\":0.190012,\"unit\":3},\"temperature\":{\"magnitude\":-0.629962,\"unit\":4},\"supply\":{\"magnitude\":1.0,\"unit\":18}},\"raw\":{\"signal\":{\"magnitude\":38.745093934,\"unit\":22},\"bridgeResistance\":{\"magnitude\":3334.3584759,\"unit\":28}},\"compensated\":{\"mathematicalModels\":{\"MM0123\":{\"pressure\":{\"output\":{\"magnitude\":0.190009,\"unit\":3},\"error\":{\"magnitude\":-0.00077952474,\"unit\":7}},\"temperature\":{\"output\":{\"magnitude\":-0.745805,\"unit\":4},\"error\":{\"magnitude\":-0.11584331,\"unit\":4}}}}}},{\"reference\":\"F_12300_XX_0000098765\",\"environmentTarget\":{\"pressure\":{\"magnitude\":0.27,\"unit\":3},\"temperature\":{\"magnitude\":0.0,\"unit\":4}},\"environment\":{\"pressure\":{\"magnitude\":0.270003,\"unit\":3},\"temperature\":{\"magnitude\":-0.629962,\"unit\":4},\"supply\":{\"magnitude\":1.0,\"unit\":18}},\"raw\":{\"signal\":{\"magnitude\":49.786859682,\"unit\":22},\"bridgeResistance\":{\"magnitude\":3330.2942637,\"unit\":28}},\"compensated\":{\"mathematicalModels\":{\"MM0123\":{\"pressure\":{\"output\":{\"magnitude\":0.270012,\"unit\":3},\"error\":{\"magnitude\":0.0025864349,\"unit\":7}},\"temperature\":{\"output\":{\"magnitude\":-0.751827,\"unit\":4},\"error\":{\"magnitude\":-0.12186504,\"unit\":4}}}}}},{\"reference\":\"F_12300_XX_0000098765\",\"environmentTarget\":{\"pressure\":{\"magnitude\":0.35,\"unit\":3},\"temperature\":{\"magnitude\":0.0,\"unit\":4}},\"environment\":{\"pressure\":{\"magnitude\":0.350001,\"unit\":3},\"temperature\":{\"magnitude\":-0.629962,\"unit\":4},\"supply\":{\"magnitude\":1.0,\"unit\":18}},\"raw\":{\"signal\":{\"magnitude\":60.782440749,\"unit\":22},\"bridgeResistance\":{\"magnitude\":3326.3508927,\"unit\":28}},\"compensated\":{\"mathematicalModels\":{\"MM0123\":{\"pressure\":{\"output\":{\"magnitude\":0.34998,\"unit\":3},\"error\":{\"magnitude\":-0.0060407687,\"unit\":7}},\"temperature\":{\"output\":{\"magnitude\":-0.753394,\"unit\":4},\"error\":{\"magnitude\":-0.12343205,\"unit\":4}}}}}},{\"reference\":\"F_12300_XX_0000098765\",\"environmentTarget\":{\"pressure\":{\"magnitude\":0.03,\"unit\":3},\"temperature\":{\"magnitude\":20.0,\"unit\":4}},\"environment\":{\"pressure\":{\"magnitude\":0.0299916,\"unit\":3},\"temperature\":{\"magnitude\":19.5509,\"unit\":4},\"supply\":{\"magnitude\":1.0,\"unit\":18}},\"raw\":{\"signal\":{\"magnitude\":17.518044987,\"unit\":22},\"bridgeResistance\":{\"magnitude\":3497.537411,\"unit\":28}},\"compensated\":{\"mathematicalModels\":{\"MM0123\":{\"pressure\":{\"output\":{\"magnitude\":0.0300046,\"unit\":3},\"error\":{\"magnitude\":0.0037184642,\"unit\":7}},\"temperature\":{\"output\":{\"magnitude\":19.5422,\"unit\":4},\"error\":{\"magnitude\":-0.0086876459,\"unit\":4}}}}}},{\"reference\":\"F_12300_XX_0000098765\",\"environmentTarget\":{\"pressure\":{\"magnitude\":0.11,\"unit\":3},\"temperature\":{\"magnitude\":20.0,\"unit\":4}},\"environment\":{\"pressure\":{\"magnitude\":0.109995,\"unit\":3},\"temperature\":{\"magnitude\":19.5509,\"unit\":4},\"supply\":{\"magnitude\":1.0,\"unit\":18}},\"raw\":{\"signal\":{\"magnitude\":28.627677565,\"unit\":22},\"bridgeResistance\":{\"magnitude\":3493.3028946,\"unit\":28}},\"compensated\":{\"mathematicalModels\":{\"MM0123\":{\"pressure\":{\"output\":{\"magnitude\":0.10997,\"unit\":3},\"error\":{\"magnitude\":-0.007028402,\"unit\":7}},\"temperature\":{\"output\":{\"magnitude\":19.5356,\"unit\":4},\"error\":{\"magnitude\":-0.015274724,\"unit\":4}}}}}},{\"reference\":\"F_12300_XX_0000098765\",\"environmentTarget\":{\"pressure\":{\"magnitude\":0.19,\"unit\":3},\"temperature\":{\"magnitude\":20.0,\"unit\":4}},\"environment\":{\"pressure\":{\"magnitude\":0.189994,\"unit\":3},\"temperature\":{\"magnitude\":19.5509,\"unit\":4},\"supply\":{\"magnitude\":1.0,\"unit\":18}},\"raw\":{\"signal\":{\"magnitude\":39.710129115,\"unit\":22},\"bridgeResistance\":{\"magnitude\":3489.1859301,\"unit\":28}},\"compensated\":{\"mathematicalModels\":{\"MM0123\":{\"pressure\":{\"output\":{\"magnitude\":0.190007,\"unit\":3},\"error\":{\"magnitude\":0.003608738,\"unit\":7}},\"temperature\":{\"output\":{\"magnitude\":19.5348,\"unit\":4},\"error\":{\"magnitude\":-0.016090891,\"unit\":4}}}}}},{\"reference\":\"F_12300_XX_0000098765\",\"environmentTarget\":{\"pressure\":{\"magnitude\":0.27,\"unit\":3},\"temperature\":{\"magnitude\":20.0,\"unit\":4}},\"environment\":{\"pressure\":{\"magnitude\":0.269996,\"unit\":3},\"temperature\":{\"magnitude\":19.5509,\"unit\":4},\"supply\":{\"magnitude\":1.0,\"unit\":18}},\"raw\":{\"signal\":{\"magnitude\":50.752763545,\"unit\":22},\"bridgeResistance\":{\"magnitude\":3485.1042867,\"unit\":28}},\"compensated\":{\"mathematicalModels\":{\"MM0123\":{\"pressure\":{\"output\":{\"magnitude\":0.270026,\"unit\":3},\"error\":{\"magnitude\":0.0086455755,\"unit\":7}},\"temperature\":{\"output\":{\"magnitude\":19.5292,\"unit\":4},\"error\":{\"magnitude\":-0.021720532,\"unit\":4}}}}}},{\"reference\":\"F_12300_XX_0000098765\",\"environmentTarget\":{\"pressure\":{\"magnitude\":0.35,\"unit\":3},\"temperature\":{\"magnitude\":20.0,\"unit\":4}},\"environment\":{\"pressure\":{\"magnitude\":0.350005,\"unit\":3},\"temperature\":{\"magnitude\":19.5509,\"unit\":4},\"supply\":{\"magnitude\":1.0,\"unit\":18}},\"raw\":{\"signal\":{\"magnitude\":61.752720945,\"unit\":22},\"bridgeResistance\":{\"magnitude\":3481.1270046,\"unit\":28}},\"compensated\":{\"mathematicalModels\":{\"MM0123\":{\"pressure\":{\"output\":{\"magnitude\":0.350005,\"unit\":3},\"error\":{\"magnitude\":-4.953976E-06,\"unit\":7}},\"temperature\":{\"output\":{\"magnitude\":19.527,\"unit\":4},\"error\":{\"magnitude\":-0.023852919,\"unit\":4}}}}}},{\"reference\":\"F_12300_XX_0000098765\",\"environmentTarget\":{\"pressure\":{\"magnitude\":0.03,\"unit\":3},
